vi "Fetch Set-Point Driver Message.vi"() -> (0 "Timed Out":bool, 1 "Message":T1)   [LabVIEW 2013]
uses:
  Set-Point Driver Messages.ctl
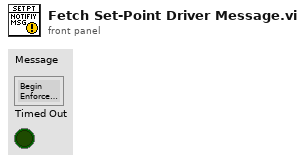
[diagram p1: front panel]
types:
  T1 = typedef "Set-Point Driver Messages.ctl" = enum16{"Begin Enforcement", "Cease Enforcement"}
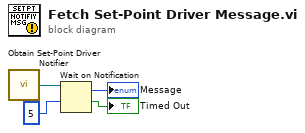
[diagram p0: block diagram]
diagram:
  n1 = call "Obtain Set-Point Driver Notifier.vi"() -> ("Set-Point Driver Notifier"=w4:refnum<notifier>)
  n2 = Wait on Notification(notifier=w4, timeout in ms (-1)=5) -> (notification=→"Message":T1, timed out?=→"Timed Out":bool)  [unwired: 2 in, 2 out]
